vi "Rx Message to Transfer Handle - BC.vi"(8 "error in":errorcluster, 9 "message":T2={"name"="", "message type"="BC to RT", "endpoint Tx"={"terminal address"=0, "subaddress"=0}, "endpoint Rx"={"terminal address"=0, "subaddress"=0}, "create timestamp channel"=FALSE, "mode code"=0, "number of words"=0, "parameters"=[]}, 11 "bus controller handle":u64) -> (0 "error out":errorcluster, 2 "valid?":bool, 3 "Rx read info":T1)   [LabVIEW 2020, in "AIM MIL-STD-1553 Engine.lvlib" / "Implementation.lvlib" / "Rx Execution Unit.lvclass"]
uses:
  Rx Execution Unit.lvclass
  <instrlib>/BTI1553Lib/BTI1553LV.lvlib
  Shared/Address.ctl
  Shared/Rx Read Info.ctl
  Shared/Terminal Endpoint.ctl
  Shared/Parameter Definition.ctl
  Shared/Message Type.ctl
  Shared/Message Definition.ctl
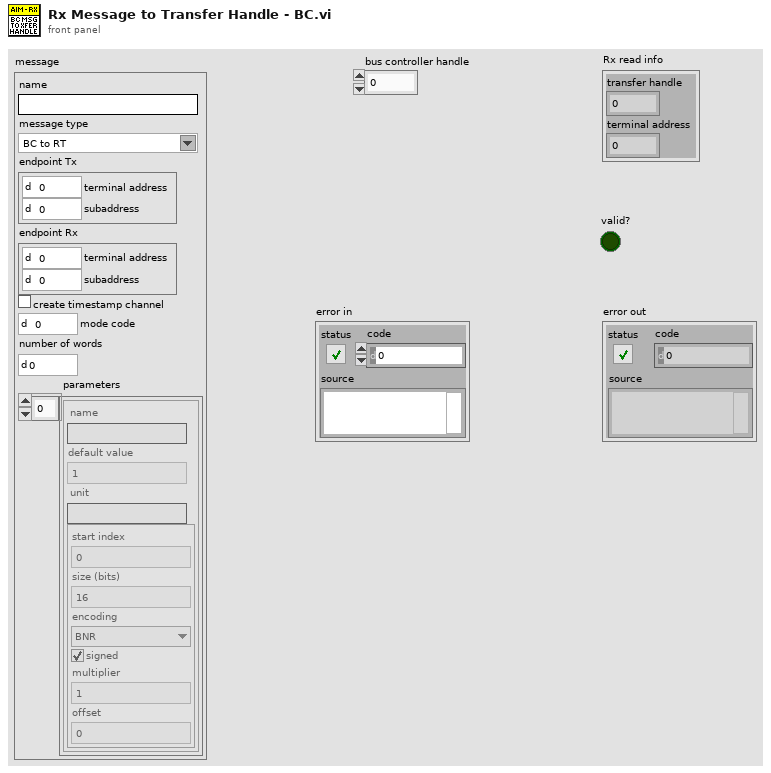
[diagram p1: front panel]
types:
  T1 = typedef "Rx Read Info.ctl" = cluster{"transfer handle":u64, "terminal address":u16}
  T2 = typedef "Message Definition.ctl" = cluster{"name":string, "message type":T3, "endpoint Tx":T4, "endpoint Rx":T4, "create timestamp channel":bool, "mode code":u16, "number of words":u16, "parameters":cluster{"name":string, "default value":dbl, "unit":string, "parameter definition":T6}[]}
  T3 = typedef "Message Type.ctl" = string
  T4 = typedef "Terminal Endpoint.ctl" = cluster{"terminal address":T5, "subaddress":T5}
  T5 = typedef "Address.ctl" = u16
  T6 = typedef "Parameter Definition.ctl" = cluster{"start index":i32, "size (bits)":i32, "encoding":enum16{"BNR", "BCD", "Discrete"}, "signed":bool, "multiplier":dbl, "offset":dbl}
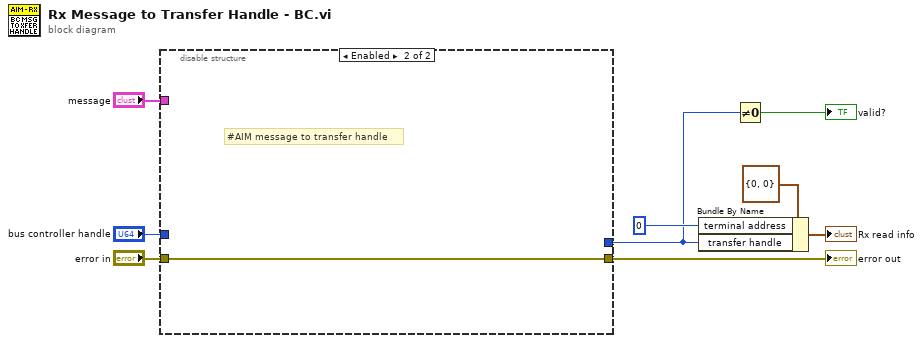
[diagram p0: block diagram]
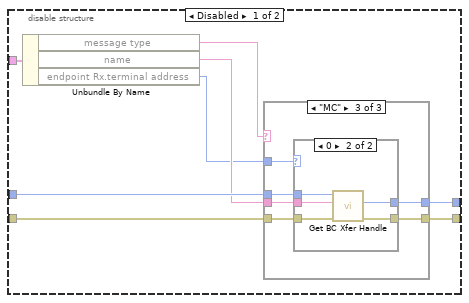
[diagram p2: hidden frame]
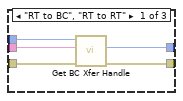
[diagram p3: hidden frame]
diagram:
  n1 = disable-structure shown="Enabled" {
    disable-tunnel: "message" -> [w17 _]
    disable-tunnel: "error in" -> [w16 w36]
    disable-tunnel: [w15 w36] -> w7
    disable-tunnel: "bus controller handle" -> [w14 _]
    disable-tunnel: [w13 _] -> w1
    frame Disabled {
      n2 = Unbundle By Name(w17) -> ("message type"=w10:T3, "name"=w12:string, "endpoint Rx.terminal address"=w11:T5)
      n3 = case shown="\"MC\"" w10 {
        tunnel: w16 -> [w22 w23 w29]
        tunnel: [w21 w23 w28] -> w15
        tunnel: w14 -> [w18 _ w27]
        tunnel: [w20 _ w26] -> w13
        tunnel: w12 -> [w19 _ w25]
        tunnel: w11 -> [_ _ w24]
        frame "RT to BC", "RT to RT" {
          n4 = call <instrlib>:"Get BC Xfer Handle.vi"("error in (no error)"=w22, "bc transfer name"=w19, "bus controller handle in"=w18) -> ("error out"=w21:errorcluster, "bc transfer handle out"=w20:u64)  [unwired: 6 in, 1 out]
        }
        frame "BC to RT", Default {
        }
        frame "MC" {
          n5 = case shown="0" w24 {
            tunnel: w29 -> [w30 w35]
            tunnel: [w30 w34] -> w28
            tunnel: w27 -> [_ w33]
            tunnel: [_ w32] -> w26
            tunnel: w25 -> [_ w31]
            frame Default {
            }
            frame 0 {
              n6 = call <instrlib>:"Get BC Xfer Handle.vi"("error in (no error)"=w35, "bc transfer name"=w31, "bus controller handle in"=w33) -> ("error out"=w34:errorcluster, "bc transfer handle out"=w32:u64)  [unwired: 6 in, 1 out]
            }
          }
        }
      }
    }
    frame Enabled {
      # "#AIM message to transfer handle"
    }
  }
  "error out" <- w7
  n7 = Bundle By Name(cluster=T1 {"transfer handle"=0, "terminal address"=0} ("Rx read info"), "terminal address"=T5 0, "transfer handle"=w1) -> (→"Rx read info":T1)
  n8 = Not Equal To 0?(x=w1) -> (x != 0?=→"valid?":bool)
